vi "Read Engine Setting.vi"(8 "error in (no error)":errorcluster, 11 "Engine configuration in":refnum<class "Engine configuration.lvclass">) -> (0 "error out":errorcluster, 2 "Engine Setting":T1={"Enabled"=TRUE, "IP Address"="127.0.0.1", "Port"=3331, "Description"="Type = Class \n", "Type"="none", "Version"="1.0.0.0"}, 3 "Engine configuration out":refnum<class "Engine configuration.lvclass">)   [LabVIEW 2025, in "Abstract Engine.lvlib" / "Engine configuration.lvclass"]
uses:
  Engine configuration.lvclass
  Engine Setting.ctl
  Engine configuration.lvclass/Engine configuration.ctl
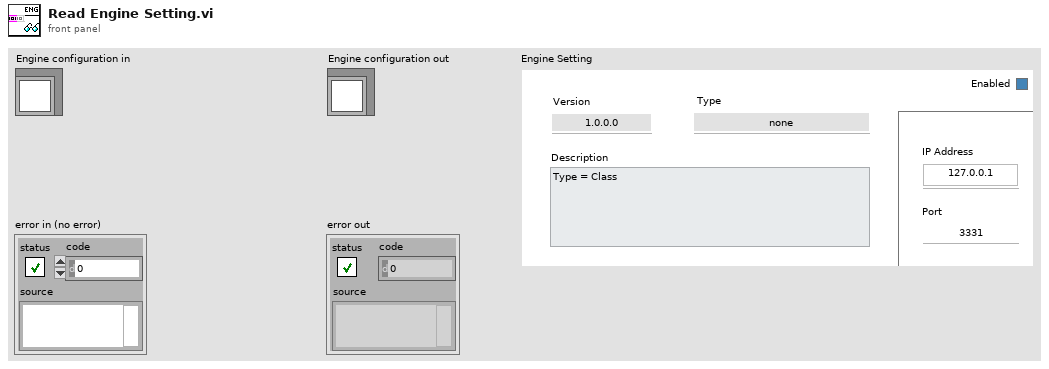
[diagram p1: front panel]
types:
  T1 = typedef "Abstract Engine.lvlib/Engine configuration.lvclass/Engine Setting.ctl" = cluster{"Enabled":bool, "IP Address":string, "Port":i32, "Description":string, "Type":string, "Version":string}
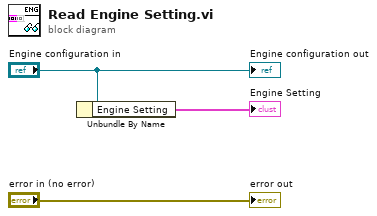
[diagram p0: block diagram]
diagram:
  n1 = Unbundle By Name("Engine configuration in") -> ("Engine Setting"=→"Engine Setting":T1)
  "error out" <- "error in (no error)"
  "Engine configuration out" <- "Engine configuration in"
